vi "b36_to_number.vi"(1 "Base36 string":string) -> (0 "Number":i32)   [LabVIEW 2023]
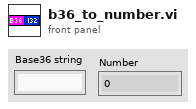
[diagram p1: front panel]
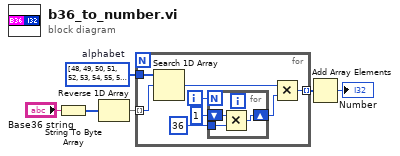
[diagram p0: block diagram]
diagram:
  w5 = u8[] [48, 49, 50, 51, 52, 53, 54, 55, 56, 57, 97, 98, 99, 100, 101, 102, 103, 104, 105, 106, 107, 108, 109, 110, 111, 112, 113, 114, 115, 116, 117, 118, 119, 120, 121, 122]  # alphabet
  n1 = String To Byte Array(string="Base36 string") -> (unsigned byte array=w1:u8[])
  n2 = Reverse 1D Array(array=w1) -> (reversed array=w6:u8[])
  n3 = for {
    tunnel: w6 -> [w13] mode=indexing
    tunnel: w5 -> [w14]
    tunnel: [w7] -> w4 mode=indexing
    i -> [w12]
    n4 = Search 1D Array(1D array=w14, element=w13) -> (index of element=w11:i32)  [unwired: 1 in]
    n5 = for {
      N: w12 -> [_]
      shift-right: [w15] -> w9
      shift-left: 1 -> [w17]
      tunnel: 36 ("y") -> [w16]
      n6 = Multiply(x=w17, y=w16) -> (x*y=w15:i32)
    }
    n7 = Multiply(x=w11, y=w9) -> (x*y=w7:i32)
  }
  n8 = Add Array Elements(numeric array=w4) -> (sum=→"Number":i32)
